vi "Requests To Table.vi"(7 "Image Folder Path":path, 10 "List Default Event":bool, 11 "Dqmh Events":refnum<class "Vi.lvclass">[](array[class])) -> (3 "Table":refnum<class "Bloc.lvclass">[](array[class]))   [LabVIEW 2021, in "TAF Proj Document Type.lvlib" / "Dqmh Module.lvclass"]
uses:
  <vilib>/Wovalab/AntiDoc/Document Type/Add-ons/LabVIEW TAF Project/Dqmh Module/Dqmh Module.lvclass
  <vilib>/Wovalab/AntiDoc/Document Type/Add-ons/LabVIEW TAF Project/Vi/Vi.lvclass
  <vilib>/Wovalab/AsciiDoc for LabVIEW/Adoc-Bloc/Bloc.lvclass
  <vilib>/Wovalab/AsciiDoc for LabVIEW/Table/Table Attributes--cluster.ctl
  <vilib>/Wovalab/AsciiDoc for LabVIEW/Table/Frame--enum.ctl
  <vilib>/Wovalab/AsciiDoc for LabVIEW/Table/Grid--enum.ctl
  <vilib>/Wovalab/AsciiDoc for LabVIEW/Table/Stripes--enum.ctl
  <vilib>/Wovalab/AsciiDoc for LabVIEW/Table/Column Attributes--cluster.ctl
  <vilib>/Wovalab/AsciiDoc for LabVIEW/Table/Horizontal Alignment--enum.ctl
  <vilib>/Wovalab/AsciiDoc for LabVIEW/Table/Vertical Alignment--enum.ctl
  <vilib>/Wovalab/AsciiDoc for LabVIEW/Table/Style--enum.ctl
  <vilib>/Wovalab/AsciiDoc for LabVIEW/Admonition/Types--enum.ctl
  <vilib>/Wovalab/AntiDoc/Document Type/Add-ons/LabVIEW TAF Project/Dqmh Event/Dqmh Event.lvclass
  C:/Program Files (x86)/National Instruments/LabVIEW 2021/vi.lib/Wovalab/AntiDoc/Bloc/Bloc.lvclass
  C:/Program Files (x86)/National Instruments/LabVIEW 2021/vi.lib/Wovalab/AntiDoc/Document Type/Add-ons/LabVIEW TAF Project/Vi/Vi.lvclass
  <vilib>/Wovalab/AntiDoc/Bloc/Bloc.lvclass/Bloc.ctl
  <vilib>/Wovalab/AntiDoc/Document Type/Add-ons/LabVIEW TAF Project/Dqmh Event/Dqmh Event.lvclass/Dqmh Event.ctl
  <vilib>/Wovalab/AntiDoc/Document Type/Add-ons/LabVIEW TAF Project/Vi/Vi.lvclass/Vi.ctl
  <vilib>/Wovalab/AsciiDoc for LabVIEW/Table/Table.lvclass/Table.ctl
  <vilib>/Wovalab/AntiDoc/Bloc/Read Name.vi
  <vilib>/Wovalab/AntiDoc/Document Type/Add-ons/LabVIEW TAF Project/Dqmh Event/Read Event Type.vi
  <vilib>/Wovalab/AntiDoc/Document Type/Add-ons/LabVIEW TAF Project/Vi/Read Conpane Image.vi
  <vilib>/Wovalab/AntiDoc/Document Type/Add-ons/LabVIEW TAF Project/Vi/Read Description.vi
  <vilib>/Wovalab/AntiDoc/Document Type/Add-ons/LabVIEW TAF Project/Vi/Read Is Reentrant.vi
  <vilib>/Wovalab/AntiDoc/Document Type/Add-ons/LabVIEW TAF Project/Vi/Read Reentrancy Type.vi
  <vilib>/Wovalab/AntiDoc/Document Type/Add-ons/LabVIEW TAF Project/Vi/Read Inline SubVI.vi
  <vilib>/Wovalab/AntiDoc/Document Type/Add-ons/LabVIEW TAF Project/Vi/Read Access Scope.vi
  <vilib>/Wovalab/AsciiDoc for LabVIEW/Table/Table.lvclass
  C:/Program Files (x86)/National Instruments/LabVIEW 2021/vi.lib/Wovalab/AsciiDoc for LabVIEW/Adoc-Bloc/Bloc.lvclass
  <vilib>/Wovalab/AsciiDoc for LabVIEW/Paragraph/Paragraph.lvclass
  <vilib>/Wovalab/AsciiDoc for LabVIEW/Admonition/Admonition.lvclass
  <vilib>/Wovalab/Asciidoc for LabVIEW/Image/Image.lvclass
  <vilib>/Wovalab/AntiDoc/Utilities/Utilities.lvlib
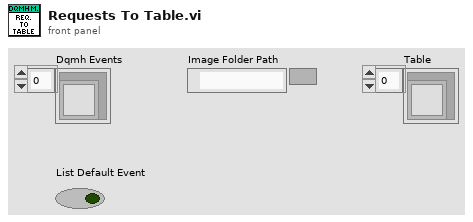
[diagram p1: front panel]
types:
  T1 = typedef "Wovalab_lib_AsciiDoctor.lvlib/Admonition.lvclass/Types--enum.ctl" = enum16{"Note", "Tip", "Important", "Warning", "Caution"}
  T2 = typedef "Wovalab_lib_AsciiDoctor.lvlib/Table.lvclass/Column Attributes--cluster.ctl" = cluster{"Width":u16, "Horizontal Alignment":T3, "Vertical Alignment":T4, "Style":T5}
  T3 = typedef "Wovalab_lib_AsciiDoctor.lvlib/Table.lvclass/Horizontal Alignment--enum.ctl" = enum16{"Left", "Center", "Right"}
  T4 = typedef "Wovalab_lib_AsciiDoctor.lvlib/Table.lvclass/Vertical Alignment--enum.ctl" = enum16{"Top", "Middle", "Bottom"}
  T5 = typedef "Wovalab_lib_AsciiDoctor.lvlib/Table.lvclass/Style--enum.ctl" = enum16{"None", "AsciiDoc", "Emphasis", "Header", "Literal", "Monospaced", "Strong", "Verse"}
  T6 = typedef "Wovalab_lib_AsciiDoctor.lvlib/Table.lvclass/Table Attributes--cluster.ctl" = cluster{"autowidth":bool, "Witdth":u8, "Frame":T7, "Grid":T8, "Stripes":T9}
  T7 = typedef "Wovalab_lib_AsciiDoctor.lvlib/Table.lvclass/Frame--enum.ctl" = enum16{"all", "topbot", "sides", "none"}
  T8 = typedef "Wovalab_lib_AsciiDoctor.lvlib/Table.lvclass/Grid--enum.ctl" = enum16{"all", "rows", "cols", "none"}
  T9 = typedef "Wovalab_lib_AsciiDoctor.lvlib/Table.lvclass/Stripes--enum.ctl" = enum16{"none", "even", "odd", "all", "hover"}
  T10 = typedef "TAF Proj Document Type.lvlib/Project Parser.lvlib/Dqmh Event Type--enum.ctl" = enum16{"Not a DQMH Event", "Request", "Request And Wait For Reply", "Broadcast"}
  T11 = typedef "imagedata.ctl" = cluster{"image type":i32, "image depth":i32, "image":u8[], "mask":u8[], "colors":u32[], "Rectangle":cluster{"left":i16, "top":i16, "right":i16, "bottom":i16}}
  T12 = enum16{"Share clones between instances", "Preallocate clone for each instance"}
  T13 = enum32{"invalid scope", "public", "private", "protected", "community"}
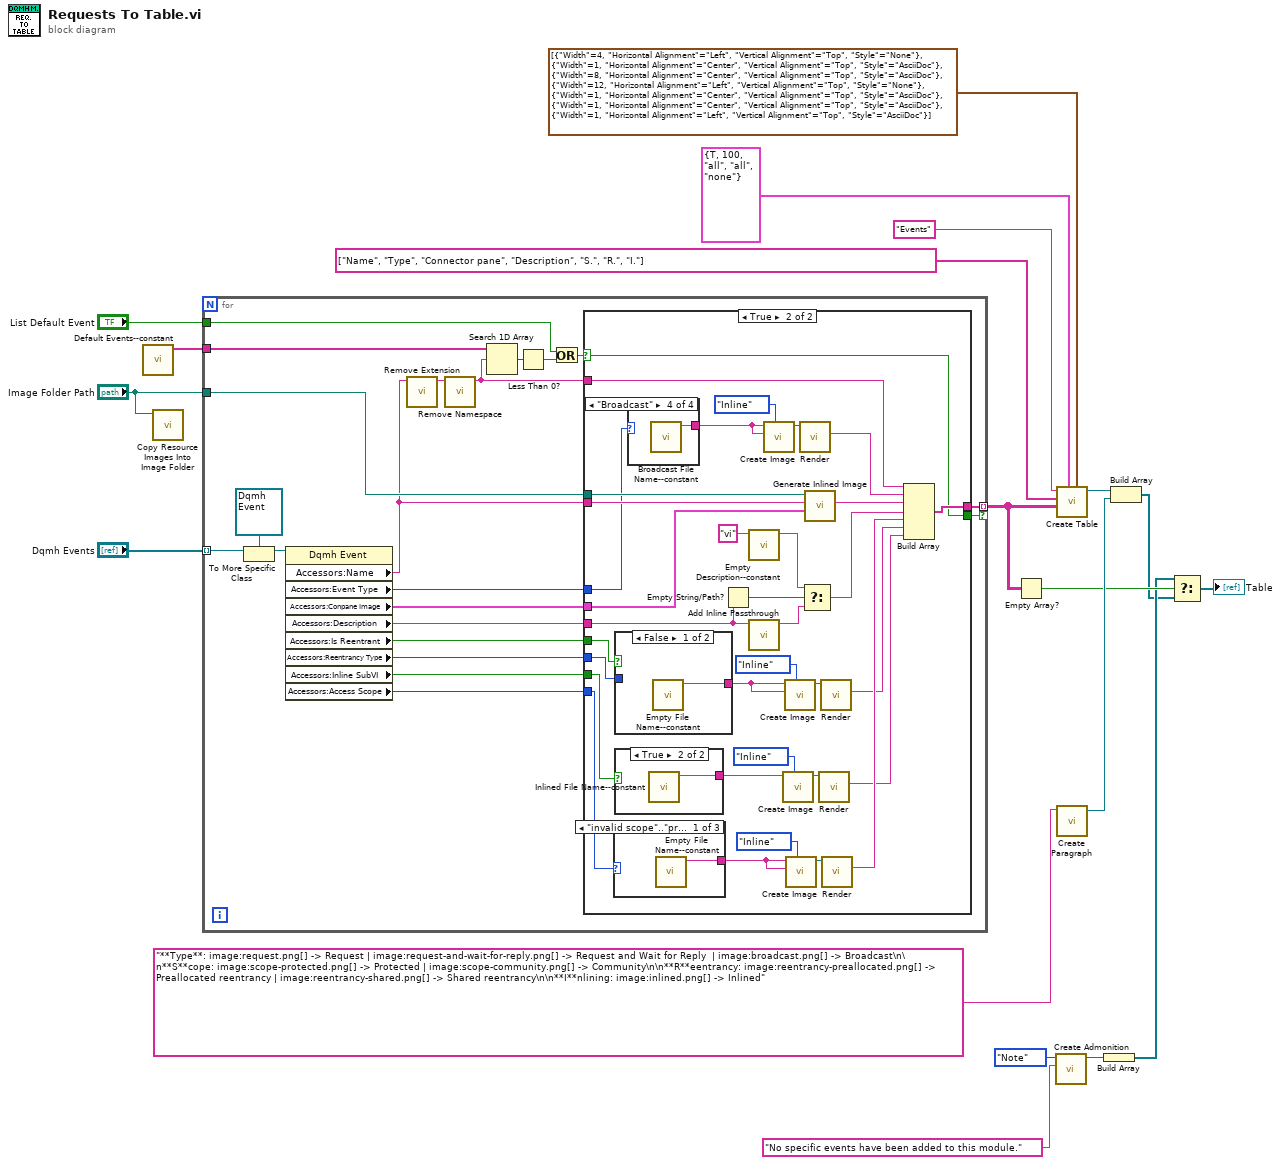
[diagram p0: block diagram]
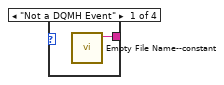
[diagram p3: hidden frame]
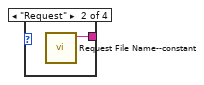
[diagram p4: hidden frame]
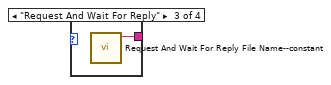
[diagram p5: hidden frame]
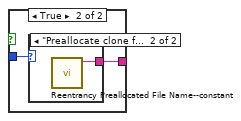
[diagram p6: hidden frame]
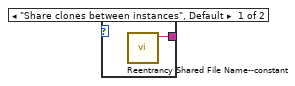
[diagram p7: hidden frame]
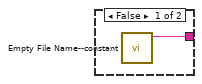
[diagram p8: hidden frame]
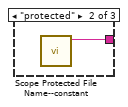
[diagram p9: hidden frame]
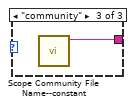
[diagram p10: hidden frame]
diagram:
  n1 = call <vilib>:"Default Events--constant.vi"() -> ("Default Event Names"=w11:string[])  [unwired: 11 in]
  n2 = call <vilib>:"Copy Resource Images Into Image Folder.vi"("Image Folder Path"="Image Folder Path") -> ()  [unwired: 9 in, 2 out]
  n3 = for {
    tunnel: "Dqmh Events" -> [w38] mode=indexing
    tunnel: "Image Folder Path" -> [w39]
    tunnel: [w40] -> w7 mode=indexing if=w25
    tunnel: w11 -> [w28]
    tunnel: "List Default Event" -> [w23]
    n4 = To More Specific Class(target class=refnum<class "Dqmh Event.lvclass"> refnum ("Antidoc:Dqmh Event"), reference=w38) -> (specific class reference=w32:refnum<class "Dqmh Event.lvclass">)  [unwired: 1 in, 1 out]
    n5 = property class="Dqmh Event"(reference=w32) -> ("Accessors:Name"=w22:string, "Accessors:Event Type"=w30:T10, "Accessors:Conpane Image"=w37:T11, "Accessors:Description"=w29:string, "Accessors:Is Reentrant"=w36:bool, "Accessors:Reentrancy Type"=w35:T12, "Accessors:Inline SubVI"=w34:bool, "Accessors:Access Scope"=w33:T13)  [unwired: 1 in, 2 out]
    n6 = call <vilib>:"Remove Extension.vi"("File Name"=w22) -> ("File Name Without Extension"=w21:string)  [unwired: 10 in]
    n7 = call <vilib>:"Remove Namespace.vi"("Vi Name"=w21) -> ("Vi Name Without Namespace"=w20:string)  [unwired: 10 in]
    n8 = Search 1D Array(1D array=w28, element=w20) -> (index of element=w27:i32)  [unwired: 1 in]
    n9 = Less Than 0?(x=w27) -> (x < 0?=w26:bool)
    n10 = Or(x=w23, y=w26) -> (x .or. y?=w24:bool)
    n11 = case shown="True" w24 {
      selector: w24 -> [w41 w51]
      tunnel: [_ w75] -> w40
      tunnel: w39 -> [_ w74]
      tunnel: w22 -> [_ w58]
      tunnel: w37 -> [_ w57]
      tunnel: w36 -> [_ w56]
      tunnel: w35 -> [_ w55]
      tunnel: w34 -> [_ w54]
      tunnel: w33 -> [_ w53]
      tunnel: w30 -> [_ w50]
      tunnel: w29 -> [_ w43]
      tunnel: w20 -> [_ w52]
      tunnel: [w41 w51] -> w25
      frame False {
      }
      frame True {
        n12 = case shown="\"invalid scope\"..\"private\"" w53 {
          tunnel: [w87 w88 w89] -> w70
          frame "invalid scope".."private" {
            n13 = call <vilib>:"Empty File Name--constant.vi"() -> ("Image File Name"=w87:string)  [unwired: 11 in]
          }
          frame "protected" {
            n14 = call <vilib>:"Scope Protected File Name--constant.vi"() -> ("Image File Name"=w88:string)  [unwired: 11 in]
          }
          frame "community" {
            n15 = call <vilib>:"Scope Community File Name--constant.vi"() -> ("Image File Name"=w89:string)  [unwired: 11 in]
          }
        }
        n16 = case shown="False" w56 {
          tunnel: [w80 w81] -> w64
          tunnel: w55 -> [_ w82]
          frame False {
            n17 = call <vilib>:"Empty File Name--constant.vi"() -> ("Image File Name"=w80:string)  [unwired: 11 in]
          }
          frame True {
            n18 = case shown="\"Preallocate clone for each instance\"" w82 {
              tunnel: [w83 w84] -> w81
              frame "Share clones between instances", Default {
                n19 = call <vilib>:"Reentrancy Shared File Name--constant.vi"() -> ("Image File Name"=w83:string)  [unwired: 11 in]
              }
              frame "Preallocate clone for each instance" {
                n20 = call <vilib>:"Reentrancy Preallocated File Name--constant.vi"() -> ("Image File Name"=w84:string)  [unwired: 11 in]
              }
            }
          }
        }
        n21 = case shown="True" w54 {
          tunnel: [w85 w86] -> w67
          frame False {
            n22 = call <vilib>:"Empty File Name--constant.vi"() -> ("Image File Name"=w85:string)  [unwired: 11 in]
          }
          frame True {
            n23 = call <vilib>:"Inlined File Name--constant.vi"() -> ("Image File Name"=w86:string)  [unwired: 11 in]
          }
        }
        n24 = case shown="\"Broadcast\"" w50 {
          tunnel: [w76 w77 w78 w79] -> w47
          frame "Not a DQMH Event" {
            n25 = call <vilib>:"Empty File Name--constant.vi"() -> ("Image File Name"=w76:string)  [unwired: 11 in]
          }
          frame "Request" {
            n26 = call <vilib>:"Request File Name--constant.vi"() -> ("Image File Name"=w77:string)  [unwired: 11 in]
          }
          frame "Request And Wait For Reply" {
            n27 = call <vilib>:"Request And Wait For Reply File Name--constant.vi"() -> ("Image File Name"=w78:string)  [unwired: 11 in]
          }
          frame "Broadcast" {
            n28 = call <vilib>:"Broadcast File Name--constant.vi"() -> ("Image File Name"=w79:string)  [unwired: 11 in]
          }
        }
        n29 = Empty String/Path?(string/path=w43) -> (empty?=w63:bool)
        n30 = call <vilib>:"Empty Description--constant.vi"("Description Source"="vi") -> ("Empty Description"=w44:string)  [unwired: 10 in]
        n31 = call <vilib>:"Add Inline Passthrough.vi"("String in"=w43) -> ("String out"=w42:string)  [unwired: 10 in]
        n32 = call <vilib>:"Create Image.vi"("Type"=enum16{"Block", "Inline"}."Inline", "Alt Text"=w47, "Image Path"=w47) -> ("Image out"=w49:refnum<class "Image.lvclass">)  [unwired: 7 in, 1 out]
        n33 = call <vilib>:"Create Image.vi"("Type"=enum16{"Block", "Inline"}."Inline", "Alt Text"=w67, "Image Path"=w67) -> ("Image out"=w68:refnum<class "Image.lvclass">)  [unwired: 7 in, 1 out]
        n34 = call <vilib>:"Create Image.vi"("Type"=enum16{"Block", "Inline"}."Inline", "Alt Text"=w64, "Image Path"=w64) -> ("Image out"=w66:refnum<class "Image.lvclass">)  [unwired: 7 in, 1 out]
        n35 = call <vilib>:"Create Image.vi"("Type"=enum16{"Block", "Inline"}."Inline", "Alt Text"=w70, "Image Path"=w70) -> ("Image out"=w72:refnum<class "Image.lvclass">)  [unwired: 7 in, 1 out]
        n36 = call-dynamic "Render.vi"("Adoc-Image in"=w49) -> ("Output"=w46:string)  [unwired: 8 in, 2 out]
        n37 = Select(t=w44, s=w63, f=w42) -> (s? t:f=w62:string)
        n38 = call <vilib>:"Generate Inlined Image.vi"("empty"=w57, "Name"=w58, "Image Folder Path"=w74) -> ("Image String"=w73:string)  [unwired: 6 in, 2 out]
        n39 = call-dynamic "Render.vi"("Adoc-Image in"=w68) -> ("Output"=w59:string)  [unwired: 8 in, 2 out]
        n40 = call-dynamic "Render.vi"("Adoc-Image in"=w66) -> ("Output"=w60:string)  [unwired: 8 in, 2 out]
        n41 = call-dynamic "Render.vi"("Adoc-Image in"=w72) -> ("Output"=w61:string)  [unwired: 8 in, 2 out]
        n42 = Build Array(w52, w46, w73, w62, w61, w60, w59) -> (w75:string[])
      }
    }
  }
  n43 = Empty Array?(array=w7) -> (empty?=w6:bool)
  n44 = call <vilib>:"Create Admonition.vi"("Content"="No specific events have been added to this module.", "Types"=Types--enum."Note") -> ("Admonition out"=w5:refnum<class "Admonition.lvclass">)  [unwired: 8 in, 1 out]
  n45 = call <vilib>:"Create Table.vi"("Column Attributes"=T2[] [{"Width"=4, "Horizontal Alignment"=enum."Left", "Vertical Alignment"=enum."Top", "Style"=enum."None"}, {"Width"=1, "Horizontal Alignment"=enum."Center", "Vertical Alignment"=enum."Top", "Style"=enum."AsciiDoc"}, {"Width"=8, "Horizontal Alignment"=enum."Center", "Vertical Alignment"=enum."Top", "Style"=enum."AsciiDoc"}, {"Width"=12, "Horizontal Alignment"=enum."Left", "Vertical Alignment"=enum."Top", "Style"=enum."None"}, {"Width"=1, "Horizontal Alignment"=enum."Center", "Vertical Alignment"=enum."Top", "Style"=enum."AsciiDoc"}, {"Width"=1, "Horizontal Alignment"=enum."Center", "Vertical Alignment"=enum."Top", "Style"=enum."AsciiDoc"}, {"Width"=1, "Horizontal Alignment"=enum."Left", "Vertical Alignment"=enum."Top", "Style"=enum."AsciiDoc"}], "Table Attributes"=T6 {"autowidth"=TRUE, "Witdth"=100, "Frame"=enum."all", "Grid"=enum."all", "Stripes"=enum."none"}, "Content"=w7, "Header"=string[] ["Name", "Type", "Connector pane", "Description", "S.", "R.", "I."], "Title"="Events") -> ("Table out"=w14:refnum<class "Table.lvclass">)  [unwired: 5 in, 1 out]
  n46 = call <vilib>:"Create Paragraph.vi"("Content"="**Type**: image:request.png[] -> Request | image:request-and-wait-for-reply.png[] -> Request and Wait for Reply  | image:broadcast.png[] -> Broadcast\n\n**S**cope: image:scope-protected.png[] -> Protected | image:scope-community.png[] -> Community\n\n**R**eentrancy: image:reentrancy-preallocated.png[] -> Preallocated reentrancy | image:reentrancy-shared.png[] -> Shared reentrancy\n\n**I**nlining: image:inlined.png[] -> Inlined") -> ("Paragraph out"=w12:refnum<class "Paragraph.lvclass">)  [unwired: 9 in, 1 out]
  n47 = Build Array(w5) -> (w4:refnum<class "Admonition.lvclass">[])
  n48 = Build Array(w14, w12) -> (w3:refnum<class "Bloc.lvclass">[])
  n49 = Select(t=w4, s=w6, f=w3) -> (s? t:f=→"Table":refnum<class "Bloc.lvclass">[])
